vi "String to Variant.vi"(8 "error in (no error)":errorcluster, 10 "String":string, 11 "Numeric Value in":refnum<class "Numeric Value.lvclass">) -> (0 "error out":errorcluster, 2 "Variant":variant, 3 "Numeric Value out":refnum<class "Numeric Value.lvclass">)   [LabVIEW 2020, in "Composed Columns.lvlib" / "Numeric Value.lvclass"]
uses:
  Numeric Value.lvclass
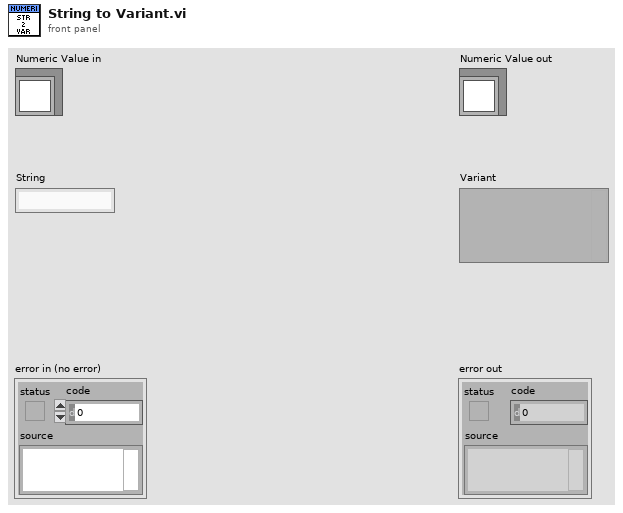
[diagram p1: front panel]
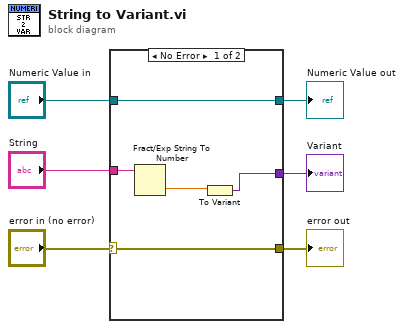
[diagram p0: block diagram]
diagram:
  n1 = case shown="No Error" "error in (no error)" {
    selector: "error in (no error)" -> [w7 w13]
    tunnel: [w7 w13] -> w5
    tunnel: "Numeric Value in" -> [w8 w12]
    tunnel: [w8 w12] -> w3
    tunnel: "String" -> [w11 _]
    tunnel: [w9 _] -> w1
    frame No Error {
      n2 = Fract/Exp String To Number(string=w11) -> (number=w10:dbl)  [unwired: 3 in, 1 out]
      n3 = To Variant(anything=w10) -> (Variant=w9:variant)
    }
    frame Error {
    }
  }
  "error out" <- w5
  "Numeric Value out" <- w3
  "Variant" <- w1
